vi "Open.vi"(8 "error in (no error)":errorcluster, 10 "address":string, 11 "Instrument.Template in":refnum<class "Instrument.Template.lvclass">) -> (0 "error out":errorcluster, 3 "Instrument.Template out":refnum<class "Instrument.Template.lvclass">)   [LabVIEW 2019, in "Instrument.Template.lvclass"]
uses:
  Instrument.Template.lvclass
  Instrument Types/VSource/Instrument.VSource.lvclass
  SMOs/Instrument/Instrument.lvclass
  C:/Users/patrick/Documents/GitHub/Instrument-Framework/lvsrc/Instrument Types/VSource/Instrument.VSource.lvclass
  C:/Users/patrick/Documents/GitHub/Instrument-Framework/lvsrc/SMOs/Instrument/Instrument.lvclass
  C:/Program Files (x86)/National Instruments/LabVIEW 2019/vi.lib/JKI/JKI SMO/SMO/SMO.lvclass
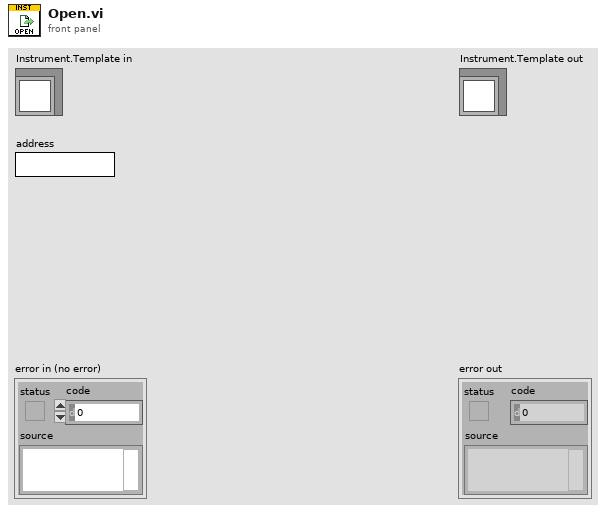
[diagram p1: front panel]
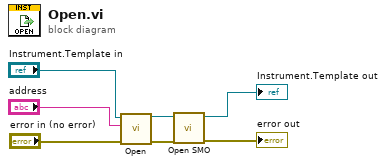
[diagram p0: block diagram]
diagram:
  n1 = call-parent "Open.vi"("error in (no error)"="error in (no error)", "address"="address", "Instrument in"="Instrument.Template in") -> ("error out"=w4:errorcluster, "Instrument out"=w3:refnum<class "Instrument.Template.lvclass">)  [unwired: 7 in]
  n2 = call "Open SMO.vi"("error in (no error)"=w4, "Instrument in"=w3) -> ("error out"=→"error out":errorcluster, "Instrument out"=→"Instrument.Template out":refnum<class "Instrument.Template.lvclass">)  [unwired: 8 in]
